vi "Programmatically Bury.vi"() -> ()   [LabVIEW 2017]
doc: "A demonstration of programmatically burying a corpse (legacy code) in a grave (Diagram Disable Structure) using the Eulogy Toolkit API. The grave is removed from the block diagram for the Bury - Simple.vi example."
uses:
  <vilib>/Utility/traverseref.llb/TRef TravTarget.ctl
  <vilib>/Utility/traverseref.llb/VI Scripting - Traverse.lvlib
  Toolkit/Toolkit.lvlib
panel:
  in  "Stop Button":bool
  # "Overview: Demonstrates programmatically burying a corpse using the Bury - Simple.vi as a target\nInstructions:\n1. Run the VI\n2. The Bury - Simple.vi's block diagram will be displayed automatically\n3. The grave will be buryed, i.e. removed from the block diagram.\n4. Click the Stop button\n5. The programmatic bury will be undone to leave the Bury - Simple.vi example in its original state."
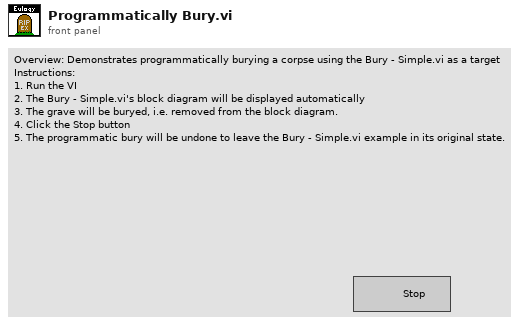
[diagram p1: front panel]
types:
  T1 = typedef "TRef TravTarget.ctl" = enum16{"FP", "BD", "Other"}
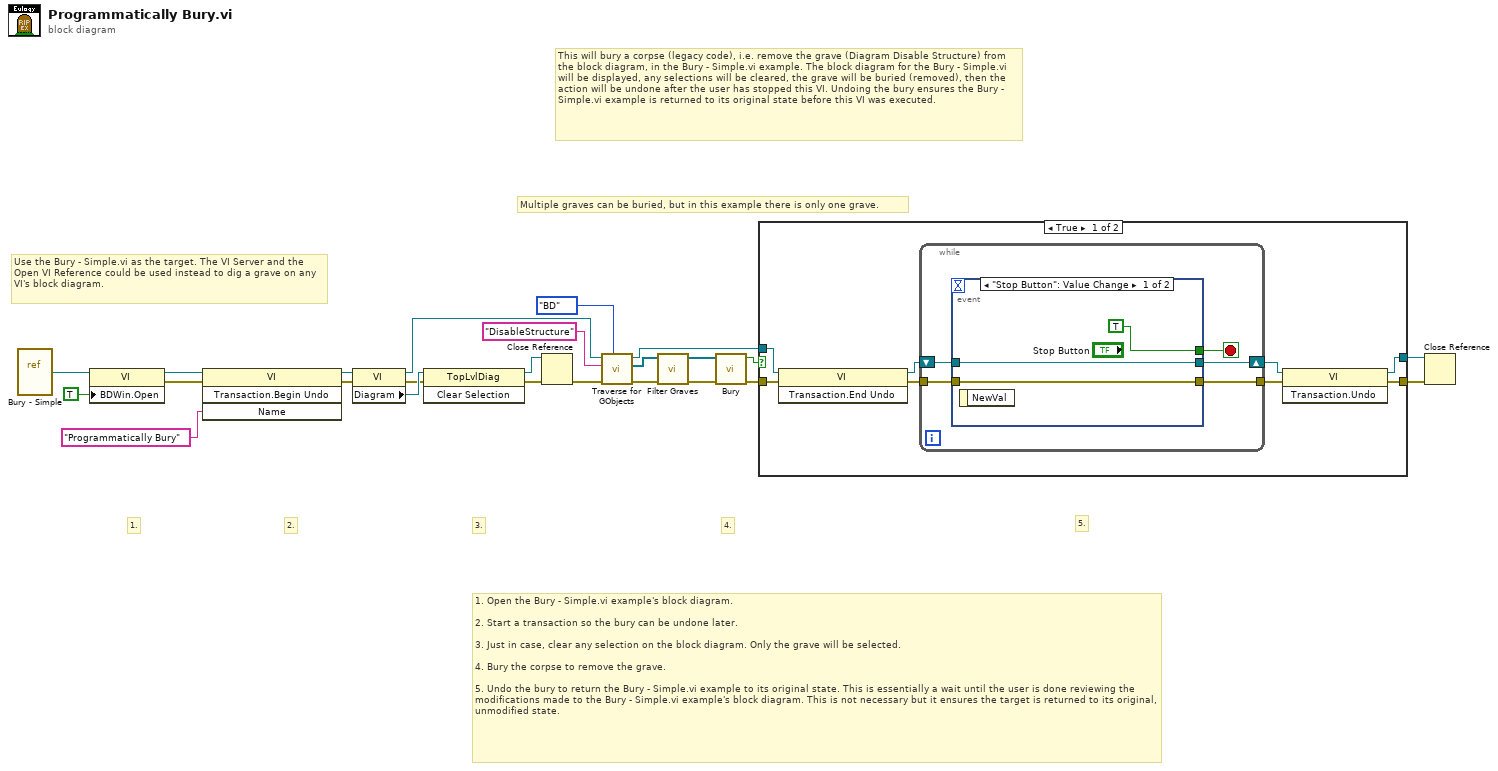
[diagram p0: block diagram]
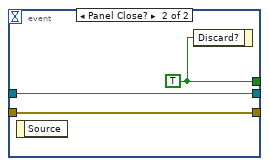
[diagram p2: hidden frame]
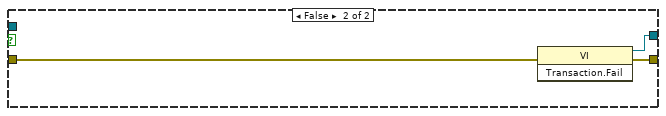
[diagram p3: hidden frame]
diagram:
  # "Multiple graves can be buried, but in this example there is only one grave."
  # "This will bury a corpse (legacy code), i.e. remove the grave (Diagram Disable Structure) from the block diagram, in the Bury - Simple.vi example. The block diagram for the Bury - Simple.vi will be displayed, any selections will be cleared, the grave will be buried (removed), then the action will be undone after the user has stopped this VI. Undoing the bury ensures the Bury - Simple.vi example is returned to its original state before this VI was executed."
  # "Use the Bury - Simple.vi as the target. The VI Server and the Open VI Reference could be used instead to dig a grave on any VI's block diagram."
  # "1. Open the Bury - Simple.vi example's block diagram.\n\n2. Start a transaction so the bury can be undone later.\n\n3. Just in case, clear any selection on the block diagram. Only the grave will be selected.\n\n4. Bury the corpse to remove the grave.\n\n5. Undo the bury to return the Bury - Simple.vi example to its original state. This is essentially a wait until the user is done reviewing the modifications made to the Bury - Simple.vi example's block diagram. This is not necessary but it ensures the target is returned to its original, unmodified state."
  # "5."
  # "4."
  # "3."
  # "2."
  # "1."
  n1 = vi-ref "Bury - Simple.vi"() -> (w20:refnum<vi>)
  n2 = property class="VI"(reference=w20, "BDWin.Open"=TRUE ("Block Diagram Window:Open")) -> (reference out=w19:refnum<vi>, error out=w17:errorcluster)  [unwired: 1 in]
  n3 = invoke class="VI" method="Transaction.Begin Undo"(reference=w19, error in=w17, "Name"="Programmatically Bury") -> (reference out=w15:refnum<vi>, error out=w14:errorcluster)  [unwired: 1 in, 2 out]
  n4 = property class="VI"(reference=w15, error in=w14) -> (reference out=w9:refnum<vi>, error out=w12:errorcluster, "Diagram"=w13:refnum<vi>)
  n5 = invoke class="TopLvlDiag" method="Clear Selection"(reference=w13, error in=w12) -> (reference out=w10:refnum<vi>, error out=w11:errorcluster)  [unwired: 1 in, 1 out]
  n6 = Close Reference(reference=w10, error in (no error)=w11) -> (error out=w8:errorcluster)
  n7 = call <vilib>:"Traverse for GObjects.vi"("Traverse Target"=TRef_TravTarget."BD", "error in (no error)"=w8, "Class Name"="DisableStructure", "VI Refnum"=w9) -> ("error out"=w4:errorcluster, "References"=w3:refnum<vi>[], "dup VI Refnum"=w7:refnum<vi>)  [unwired: 4 in, 1 out]
  n8 = call "Filter Graves.vi"("Error In"=w4, "GObjects"=w3) -> ("Error Out"=w1:errorcluster, "Graves"=w2:refnum<vi>[])  [unwired: 8 in]
  n9 = call "Bury.vi"("Error In"=w1, "Graves"=w2) -> ("Error Out"=w6:errorcluster, "Change Made?"=w5:bool)  [unwired: 8 in]
  n10 = case shown="True" w5 {
    tunnel: [w29 w46] -> w22
    tunnel: [w30 w45] -> w21
    tunnel: w7 -> [w26 _]
    tunnel: w6 -> [w25 w44]
    frame True {
      n11 = invoke class="VI" method="Transaction.End Undo"(reference=w26, error in=w25) -> (reference out=w32:refnum<vi>, error out=w28:errorcluster)  [unwired: 1 in, 1 out]
      n12 = while {
        shift-right: [w36] -> w31
        shift-left: w32 -> [w37]
        tunnel: w28 -> [w35]
        tunnel: [w34] -> w27
        stop <- w33 stop-if-true
        n13 = event shown="[0] \"Stop Button\": Value Change" {
          selector: _ -> [_ _]
          dyn-events: _ -> [_ _]
          timeout: _ -> [_ _]
          tunnel: w37 -> [w40 w43]
          tunnel: [w40 w43] -> w36
          tunnel: w35 -> [w39 w42]
          tunnel: [w39 w42] -> w34
          tunnel: [TRUE w41] -> w33
          event "Stop Button": Value Change {
            n14 = event-data() -> ()  [unwired: 1 in, 1 out]
          }
          event Panel Close? {
            w41 = TRUE
            n15 = event-data() -> ()  [unwired: 1 in, 1 out]
            n16 = event-data("Discard?"=w41) -> ()  [unwired: 1 in, 1 out]
          }
        }
      }
      n17 = invoke class="VI" method="Transaction.Undo"(reference=w31, error in=w27) -> (reference out=w30:refnum<vi>, error out=w29:errorcluster)  [unwired: 1 in, 1 out]
    }
    frame False {
      n18 = invoke class="VI" method="Transaction.Fail"(error in=w44) -> (reference out=w45:refnum<vi>, error out=w46:errorcluster)  [unwired: 2 in, 1 out]
    }
  }
  n19 = Close Reference(reference=w21, error in (no error)=w22) -> ()  [unwired: 1 out]
